vi "Save.vi"(8 "error in (no error)":errorcluster, 11 "Cluster":T2) -> (0 "error out":errorcluster)   [LabVIEW 2019]
uses:
  <vilib>/vision/Image Controls.llb/IMAQ Image.ctl
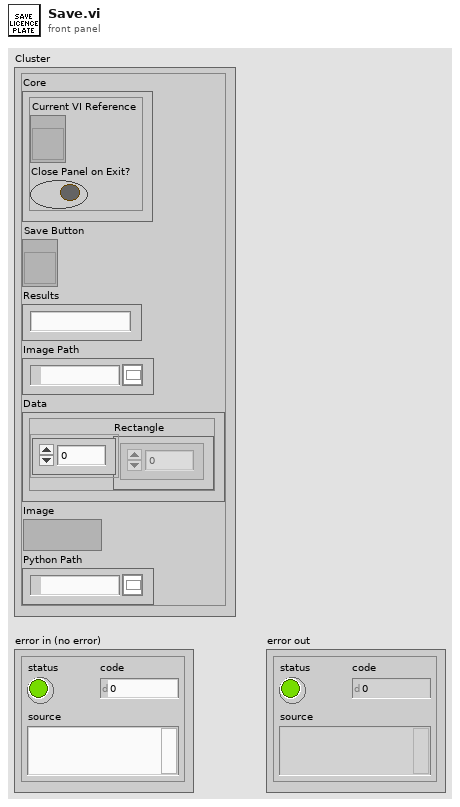
[diagram p1: front panel]
types:
  T1 = typedef "IMAQ Image.ctl" = refnum<image>
  T2 = cluster{"Core":cluster{"Current VI Reference":refnum<vi>, "Close Panel on Exit?":bool}, "Save Button":refnum<vi>, "Results":string, "Image Path":path, "Data":cluster{"Rectangle":i32[]}, "Image":T1, "Python Path":path}
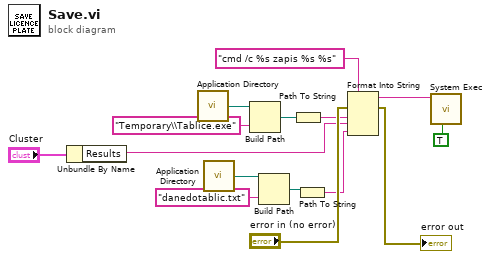
[diagram p0: block diagram]
diagram:
  n1 = Unbundle By Name("Cluster") -> ("Results"=w12:string)
  n2 = call <vilib>:"Application Directory.vi"() -> ("Application Directory"=w4:path)
  n3 = call <vilib>:"Application Directory.vi"() -> ("Application Directory"=w7:path)
  n4 = Build Path ("Tablice exe")(base path=w4, name or relative path="Temporary\\Tablice.exe") -> (appended path=w6:path)
  n5 = Build Path ("Tablice exe")(base path=w7, name or relative path="danedotablic.txt") -> (appended path=w9:path)
  n6 = Path To String(path=w6) -> (string=w11:string)
  n7 = Path To String(path=w9) -> (string=w13:string)
  n8 = Format Into String(format string="cmd /c %s zapis %s %s" ("command line"), error in="error in (no error)", w11, w12, w13) -> (resulting string=w2:string, error out=→"error out":errorcluster)  [unwired: 1 in]
  n9 = call <vilib>:"System Exec.vi"("run minimized? (F)"=TRUE, "command line"=w2) -> ()  [unwired: 6 in, 4 out]
